vi "Send StartTask.vi"(7 "Message Priority (Normal)":T1=enum."Normal", 8 "error in (no error)":errorcluster, 10 "Task":string, 11 "Message Enqueuer":refnum<class "Message Enqueuer.lvclass">) -> (0 "error out":errorcluster, 3 "Message Enqueuer out":refnum<class "Message Enqueuer.lvclass">)   [LabVIEW 2025, in "DAQ_Module.lvlib" / "StartTask Msg.lvclass"]
doc: "This VI sends the message to an actor."
uses:
  StartTask Msg.lvclass
  <vilib>/ActorFramework/Message Enqueuer/Message Enqueuer.lvclass
  <vilib>/ActorFramework/Message Enqueuer/Message Priority.ctl
  C:/Program Files (x86)/National Instruments/LabVIEW 2025/vi.lib/ActorFramework/Message/Message.lvclass
  StartTask Msg.lvclass/StartTask Msg.ctl
  <vilib>/ActorFramework/Message Enqueuer/Message Enqueuer.lvclass/Message Enqueuer.ctl
  <vilib>/ActorFramework/Message Priority Queue/Priority Enqueue.vi
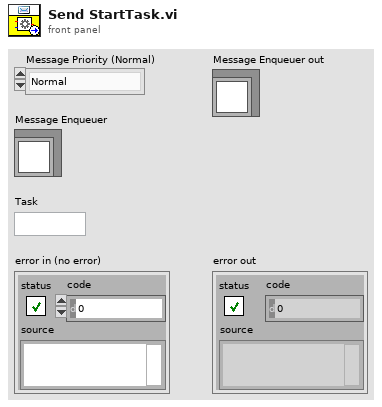
[diagram p1: front panel]
types:
  T1 = typedef "Actor Framework.lvlib/Message Enqueuer.lvclass/Message Priority.ctl" = enum16{"Low", "Normal", "High"}
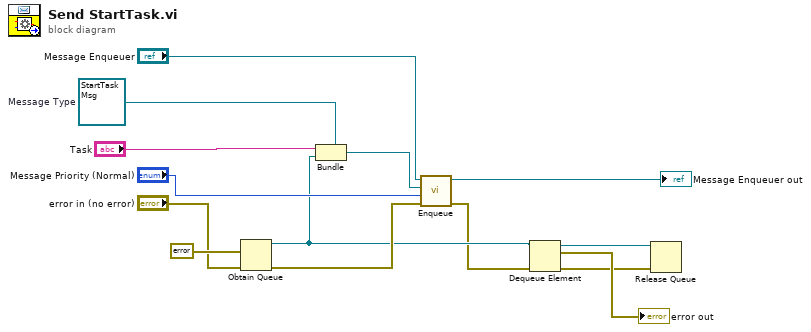
[diagram p0: block diagram]
diagram:
  w13 = refnum<class "StartTask Msg.lvclass"> refnum  # Message Type
  n1 = Obtain Queue(element data type=errorcluster {"status"=FALSE, "code"=0, "source"=""} ("error in (no error)"), error in (no error)="error in (no error)") -> (queue out=w5:refnum<queue>, error out=w6:errorcluster)  [unwired: 3 in, 1 out]
  n2 = Bundle(cluster=w13, "Task", w5) -> (w12:refnum<class "StartTask Msg.lvclass">)
  n3 = call <vilib>:"Enqueue.vi"("error in (no error)"=w6, "Message Priority (Normal)"="Message Priority (Normal)", "Message"=w12, "Message Enqueuer in"="Message Enqueuer") -> ("error out"=w4:errorcluster, "Message Enqueuer out"=→"Message Enqueuer out":refnum<class "Message Enqueuer.lvclass">)  [unwired: 6 in]
  n4 = Dequeue Element(queue=w5, error in (no error)=w4) -> (queue out=w2:refnum<queue>, element=→"error out":errorcluster, error out=w1:errorcluster)  [unwired: 1 in, 1 out]
  n5 = Release Queue(queue=w2, error in (no error)=w1) -> ()  [unwired: 1 in, 3 out]
